vi "Teleop.vi"(10 "Match Info":T2={"Autonomous Elapsed Seconds"=0.0, "TeleOp Elapsed Seconds"=0.0, "Disabled Elapsed Seconds"=0.0, "Visited Autonomous"=FALSE, "Visited TeleOp"=FALSE, "Visited Disabled"=FALSE, "Autonomous Settings"={"Autonomous Style"=enum."Independent", "VI Refnum"=refnum}}, 11 "Call Context":T3) -> ()   [LabVIEW 2020]
doc: "This VI is called for each TeleOp packet received from the DS where the robot is not disabled. It is often used to read from the joysticks and update I/O or to update setpoints for timed control loops. It should complete and return within 20 milliseconds or it may miss DS packets."
uses:
  <vilib>/Rock Robotics/WPI/DriverStation/WPI_DriverStationDerivedRobotMode.ctl
  <vilib>/Rock Robotics/WPI/DriverStation/WPI_DriverStationMatch Info.ctl
  <vilib>/Rock Robotics/WPI/Solenoid/WPI_SolenoidValue.ctl
  <vilib>/Rock Robotics/WPI/ThirdParty/Phoenix-LabVIEW/Motor Controller/Controls/CTRE_Phoenix_MotorControl_ControlMode.ctl
  <vilib>/Rock Robotics/WPI/Utilities/WPI_GetSetVariantRefNum.vi
  <vilib>/Rock Robotics/Network Tables/NT Write Boolean Array.vi
  <vilib>/Rock Robotics/Network Tables/NT Write Numeric Array.vi
  <vilib>/Rock Robotics/Network Tables/NT Read Boolean.vi
  <vilib>/Rock Robotics/Network Tables/NT Read Number.vi
  <vilib>/Rock Robotics/WPI/Solenoid/WPI_SolenoidSetEnum.vi
  Robot Global Data.vi
panel:
  out "start_control_panel":bool
  out "control_panel_arm_output":dbl
  out "encoder_setpoint":dbl=1409.0
  out "intake_motor_output":dbl
  out "control_arm_cylinder":T1
  out "intake_cylinder":T1
  out "climb_cylinder":T1
  out "Sample Slider 0":dbl(slide) scale=0.0..5.0
  out "Sample Boolean 1":bool
  out "Sample Boolean 0":bool
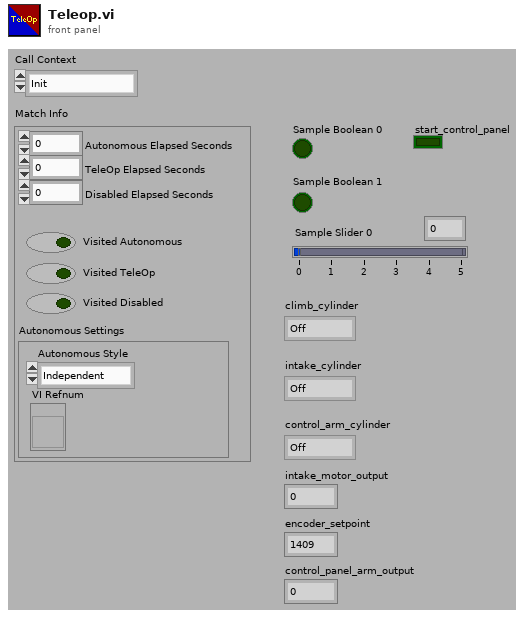
[diagram p1: front panel]
types:
  T1 = typedef "WPI_SolenoidValue.ctl" = enum16{"Off", "On", "Forward", "Reverse"}
  T2 = typedef "WPI_DriverStationMatch Info.ctl" = cluster{"Autonomous Elapsed Seconds":dbl, "TeleOp Elapsed Seconds":dbl, "Disabled Elapsed Seconds":dbl, "Visited Autonomous":bool, "Visited TeleOp":bool, "Visited Disabled":bool, "Autonomous Settings":cluster{"Autonomous Style":enum16{"Iterative", "Independent"}, "VI Refnum":refnum<vi>}}
  T3 = typedef "WPI_DriverStationDerivedRobotMode.ctl" = enum16{"Init", "Execute", "Stop"}
  T4 = typedef "CTRE_Phoenix_MotorControl_ControlMode.ctl" = u16
  T5 = typedef "WPI_JoystickDevRef.ctl" = cluster{"Device":T6}
  T6 = typedef "WPI_JoystickDeviceEnum.ctl" = enum16{"USB 0", "USB 1", "USB 2", "USB 3", "USB 4", "USB 5"}
  T7 = typedef "WPI_RobotDriveDevRef.ctl" = cluster{"DevStatus":errorcluster, "Motors[]":T8[], "Square Inputs":bool, "Max Output":dbl}
  T8 = typedef "WPI_MotorControlDeviceRef.ctl" = cluster{"DeviceStatus":errorcluster, "Type":T9, "PWM":cluster{"PWM Channel":T10, "DeadBand":T11}, "CAN":cluster{"Device Number":u8, "SetOutput VI Ref":variant, "GetOutput VI Ref":variant, "Enable VI Ref":variant, "Disable VI Ref":variant, "Data":variant}, "Invert":bool, "DIO PWM":cluster{"PWM \"Enable\" Channel":T10, "DIOChannel":T12, "PWM Rate":dbl}}
  T9 = typedef "WPI_MotorControlType.ctl" = enum16{"PWM", "CAN", "DIO PWM"}
  T10 = typedef "FPGA_DIOPWMChannel.ctl" = enum8{"PWM 0", "PWM 1", "PWM 2", "PWM 3", "PWM 4", "PWM 5", "PWM 6", "PWM 7", "PWM 8", "PWM 9", "PWM MXP 0", "PWM MXP 1", "PWM MXP 2", "PWM MXP 3", "PWM MXP 4", "PWM MXP 5", "PWM MXP 6", "PWM MXP 7", "PWM MXP 8", "PWM MXP 9", "Invalid"}
  T11 = typedef "WPI_PWMDeadband.ctl" = cluster{"Name":string, "maxPositivePwm":i32, "minPositivePwm":i32, "centerPwm":i32, "maxNegativePwm":i32, "minNegativePwm":i32, "angularRange":u16}
  T12 = typedef "FPGA_DIOChannel.ctl" = enum8{"DIO 0", "DIO 1", "DIO 2", "DIO 3", "DIO 4", "DIO 5", "DIO 6", "DIO 7", "DIO 8", "DIO 9", "DIO MXP 0", "DIO MXP 1", "DIO MXP 2", "DIO MXP 3", "DIO MXP 4", "DIO MXP 5", "DIO MXP 6", "DIO MXP 7", "DIO MXP 8", "DIO MXP 9", "DIO MXP 10", "DIO MXP 11", "DIO MXP 12", "DIO MXP 13", "DIO MXP 14", "DIO MXP 15", "SPI Port CS1", "SPI Port CS2", "SPI Port CS3", "SPI Port MISO", "SPI Port MOSI", "Invalid"}
  T13 = typedef "WPI_SolenoidDevRef.ctl" = cluster{"DevStatus":errorcluster, "Pneumatics Control Module":u8, "Forward Solenoid Channel":T14, "Reverse Solenoid Channel":T14}
  T14 = typedef "WPI_SolenoidChannel.ctl" = enum8{"Solenoid 0", "Solenoid 1", "Solenoid 2", "Solenoid 3", "Solenoid 4", "Solenoid 5", "Solenoid 6", "Solenoid 7", "Solenoid 8", "Solenoid 9", "Solenoid 10", "Solenoid 11", "Solenoid 12", "Solenoid 13", "Solenoid 14", "Solenoid 15", "Invalid"}
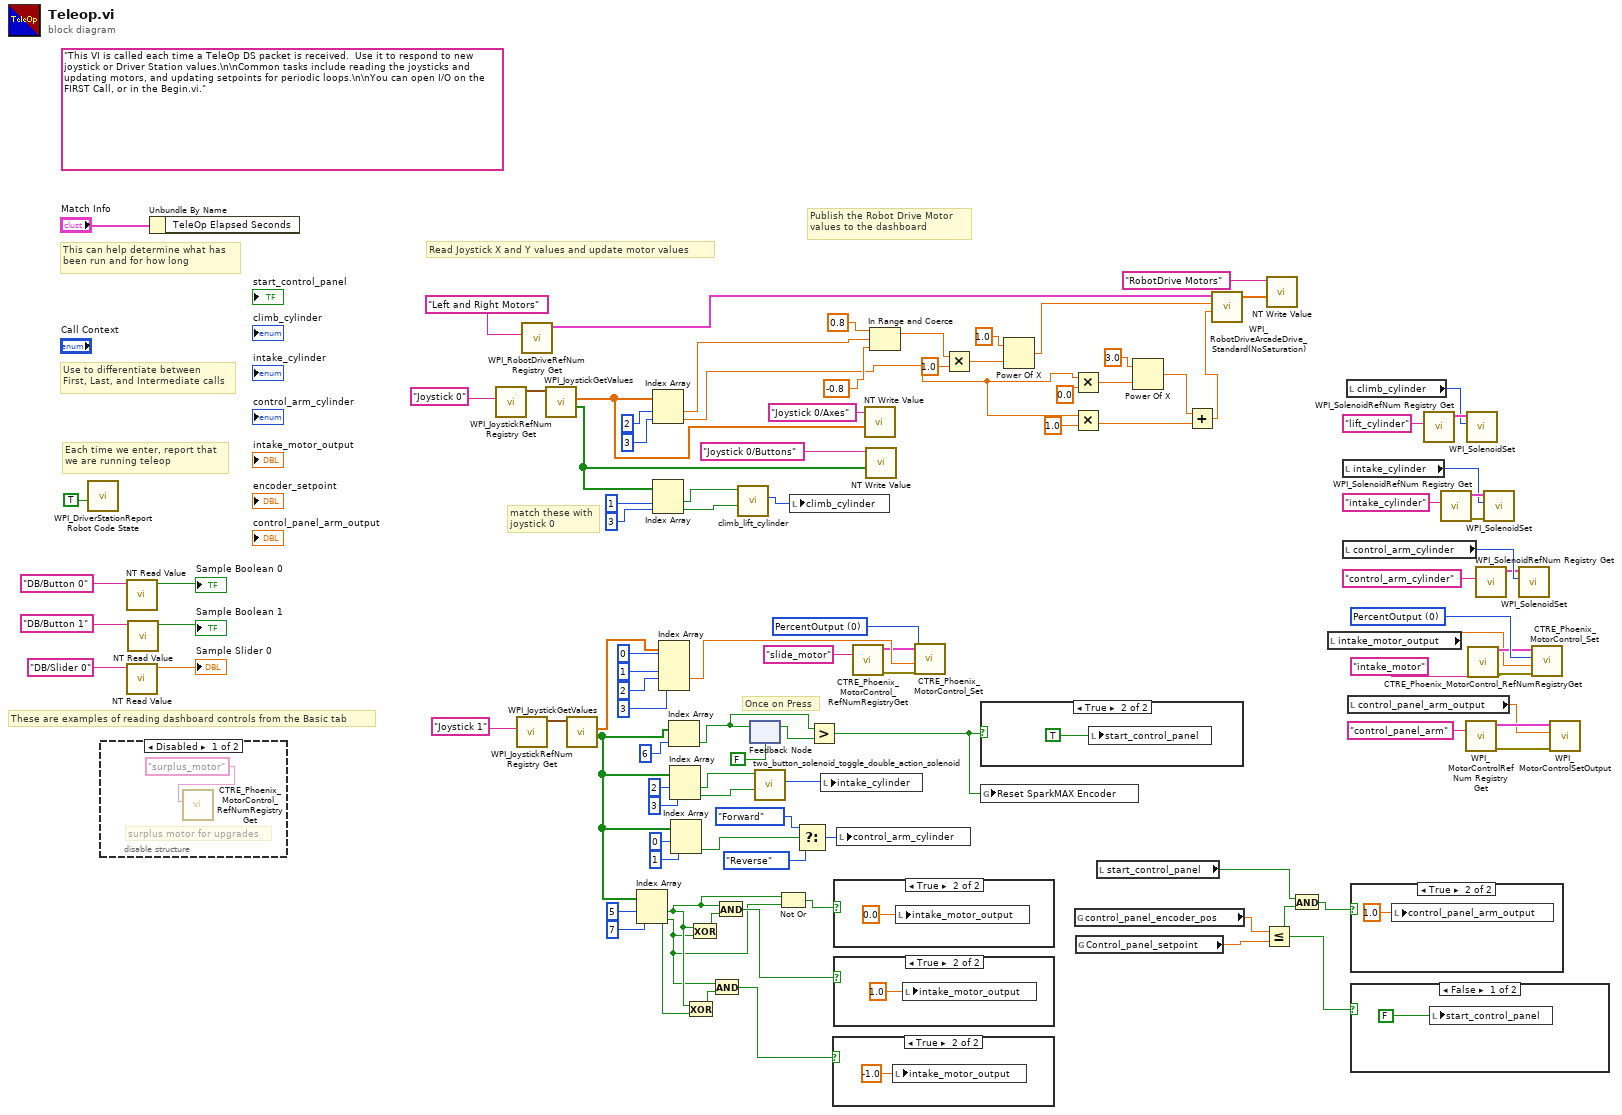
[diagram p0: block diagram]
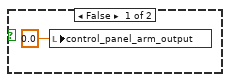
[diagram p4: hidden frame]
diagram:
  w48 = T4 0 items=["PercentOutput"=0, "Position"=1, "Velocity"=2, "Current"=3, "Follower"=5, "MotionProfile"=6, "MotionMagic"=7, "MotionProfileArc"=10, "Disabled"=15] ("Control Mode")
  w49 = T4 0 items=["PercentOutput"=0, "Position"=1, "Velocity"=2, "Current"=3, "Follower"=5, "MotionProfile"=6, "MotionMagic"=7, "MotionProfileArc"=10, "Disabled"=15] ("Control Mode")
  (unwired) "This VI is called each time a TeleOp DS packet is received.  Use it to respond to new joystick or Driver Station values.\n\nCommon tasks include reading the joysticks and updating motors, and updating setpoints for periodic loops.\n\nYou can open I/O on the FIRST Call, or in the Begin.vi."
  # "Once on Press"
  # "match these with\njoystick 0"
  # "These are examples of reading dashboard controls from the Basic tab"
  # "Publish the Robot Drive Motor\nvalues to the dashboard"
  # "Each time we enter, report that\nwe are running teleop"
  # "Use to differentiate between\nFirst, Last, and Intermediate calls"
  # "This can help determine what has\nbeen run and for how long"
  # "Read Joystick X and Y values and update motor values"
  n1 = call <vilib>:"WPI_DriverStationReport Robot Code State.vi"("TeleOp"=TRUE ("Autonomous")) -> ()  [unwired: 10 in, 1 out]
  n2 = disable-structure shown="Disabled" {
    frame Disabled {
      # "surplus motor for upgrades"
      n3 = call <vilib>:"CTRE_Phoenix_MotorControl_RefNumRegistryGet.vi"("refnum name"="surplus_motor") -> ()  [unwired: 9 in, 2 out]
    }
    frame Enabled {
    }
  }
  n4 = call-poly <vilib>:"NT Read Value.vi"("Name"="DB/Button 0" ("refnum name")) -> ("Boolean"=→"Sample Boolean 0":bool)  [unwired: 9 in, 1 out]
  n5 = call-poly <vilib>:"NT Read Value.vi"("Name"="DB/Slider 0" ("refnum name")) -> ("Numeric"=→"Sample Slider 0":dbl)  [unwired: 9 in, 1 out]
  n6 = call-poly <vilib>:"NT Read Value.vi"("Name"="DB/Button 1" ("refnum name")) -> ("Boolean"=→"Sample Boolean 1":bool)  [unwired: 9 in, 1 out]
  n7 = Unbundle By Name("Match Info") -> ()  [unwired: 1 out]
  n8 = call <vilib>:"WPI_JoystickRefNum Registry Get.vi"("refnum name"="Joystick 0") -> ("JoystickDevRef"=w99:T5)  [unwired: 1 in, 9 out]
  n9 = call <vilib>:"WPI_JoystickRefNum Registry Get.vi"("refnum name"="Joystick 1") -> ("JoystickDevRef"=w83:T5)  [unwired: 1 in, 9 out]
  n10 = call <vilib>:"WPI_RobotDriveRefNum Registry Get.vi"("refnum name"="Left and Right Motors") -> ("RobotDriveDevRef"=w101:T7)  [unwired: 1 in, 9 out]
  n11 = call <vilib>:"WPI_JoystickGetValues.vi"("JoystickDevRef"=w99) -> ("Buttons"=w81:bool[], "Axes"=w95:dbl[])  [unwired: 6 in, 3 out]
  n12 = call <vilib>:"WPI_JoystickGetValues.vi"("JoystickDevRef"=w83) -> ("Buttons"=w33:bool[], "Axes"=w84:dbl[])  [unwired: 6 in, 3 out]
  n13 = Index Array(array=w33, index #1=5 ("index"), index #2=7 ("index")) -> (element #1=w40:bool, element #2=w39:bool)
  n14 = Index Array(array=w95, index #1=2 ("index"), index #2=3 ("index")) -> (element #1=w14:dbl, element #2=w2:dbl)
  n15 = Index Array(array=w81, index #1=1 ("index"), index #2=3 ("index")) -> (element #1=w76:bool, element #2=w75:bool)
  n16 = Index Array(array=w84, index #1=0 ("index"), index #2=1 ("index"), index #3=2 ("index"), index #4=3 ("index")) -> (element #3=w56:dbl)  [unwired: 3 out]
  n17 = Index Array(array=w33, index=6) -> (element=w22:bool)
  n18 = Index Array(array=w33, index #1=2 ("index"), index #2=3 ("index")) -> (element #1=w62:bool, element #2=w61:bool)
  n19 = Index Array(array=w33, index #1=0 ("index"), index #2=1 ("index")) -> (element #2=w24:bool)  [unwired: 1 out]
  n20 = Exclusive Or(1:w39, 2:w40) -> (0:w52:bool)
  n21 = Exclusive Or(1:w39, 2:w40) -> (0:w53:bool)
  n22 = And(x=w39, y=w52) -> (x .and. y?=w50:bool)
  n23 = And(x=w40, y=w53) -> (x .and. y?=w51:bool)
  n24 = call "climb_lift_cylinder.vi"("Button A"=w76, "Button B"=w75) -> ("climb_lyft_cylinder"=w29:T1)  [unwired: 8 in]
  n25 = feedback-in #1(w22) -> ()
  n26 = feedback #1(FALSE) -> (w21:bool)
  n27 = call "two_button_solenoid_toggle_double_action_solenoid.vi"("Button A"=w62, "Button B"=w61) -> ("Cylinder_out"=w67:T1)  [unwired: 8 in]
  n28 = Not Or(1:w39, 2:w40) -> (0:w38:bool)
  n29 = local write "climb_cylinder"(w29) -> ()
  n30 = Select(t=WPI_SolenoidValue."Forward" ("Value"), s=w24, f=WPI_SolenoidValue."Reverse" ("Value")) -> (s? t:f=w27:T1)
  n31 = Greater?(x=w22, y=w21) -> (0:w17:bool)
  n32 = local write "intake_cylinder"(w67) -> ()
  n33 = case shown="True" w50 {
    frame False {
    }
    frame True {
      n34 = local write "intake_motor_output"(-1.0) -> ()
    }
  }
  n35 = case shown="True" w38 {
    frame False {
    }
    frame True {
      n36 = local write "intake_motor_output"(0.0) -> ()
    }
  }
  n37 = case shown="True" w51 {
    frame False {
    }
    frame True {
      n38 = local write "intake_motor_output"(1.0) -> ()
    }
  }
  n39 = local write "control_arm_cylinder"(w27) -> ()
  n40 = call <vilib>:"CTRE_Phoenix_MotorControl_RefNumRegistryGet.vi"("refnum name"="slide_motor") -> ("error out"=w45:errorcluster, "PhoenixMotorControlDevRef"=w46:T8)  [unwired: 9 in]
  n41 = call-poly <vilib>:"NT Write Value.vi"("Numeric Array"=w95, "Name"="Joystick 0/Axes") -> ()  [unwired: 9 in, 1 out]
  n42 = call-poly <vilib>:"NT Write Value.vi"("Boolean Array"=w81, "Name"="Joystick 0/Buttons") -> ()  [unwired: 9 in, 1 out]
  n43 = In Range and Coerce(upper limit=0.8, x=w14, lower limit=-0.8) -> (coerced(x)=w11:dbl)  [unwired: 1 out]
  n44 = call <vilib>:"CTRE_Phoenix_MotorControl_Set.vi"("error in (no error)"=w45, "Output"=w56, "Control Mode"=w48, "PhoenixMotorControlDevRef"=w46) -> ()  [unwired: 6 in, 2 out]
  n45 = Multiply(x=w11, y=1.0) -> (x*y=w10:dbl)
  n46 = case shown="True" w17 {
    frame False {
    }
    frame True {
      n47 = local write "start_control_panel"(TRUE) -> ()
    }
  }
  n48 = global write "Robot Global Data.vi" "Reset SparkMAX Encoder"(w17) -> ()
  n49 = Power Of X(1:w10, 2:1.0 ("y")) -> (0:w12:dbl)
  n50 = Multiply(x=w2, y=0.0) -> (x*y=w7:dbl)
  n51 = Multiply(x=w2, y=1.0) -> (x*y=w3:dbl)
  n52 = global read "Robot Global Data.vi" "control_panel_encoder_pos"() -> (w34:dbl)
  n53 = global read "Robot Global Data.vi" "Control_panel_setpoint"() -> (w19:dbl)
  n54 = local read "start_control_panel"() -> (w18:bool)
  n55 = Power Of X(1:w7, 2:3.0 ("y")) -> (0:w4:dbl)
  n56 = Add(x=w4, y=w3) -> (x+y=w5:dbl)
  n57 = call <vilib>:"WPI_RobotDriveArcadeDrive_Standard(NoSaturation).vi"("Y axis value"=w5, "X axis value"=w12, "RobotDriveDevRef"=w101) -> ("Motor Values"=w88:dbl[])  [unwired: 1 in, 7 out]
  n58 = Less Or Equal?(x=w34, y=w19) -> (x <= y?=w20:bool)
  n59 = call-poly <vilib>:"NT Write Value.vi"("Numeric Array"=w88, "Name"="RobotDrive Motors") -> ()  [unwired: 9 in, 1 out]
  n60 = And(x=w18, y=w20) -> (x .and. y?=w30:bool)
  n61 = local read "intake_motor_output"() -> (w41:dbl)
  n62 = local read "intake_cylinder"() -> (w70:T1)
  n63 = local read "control_arm_cylinder"() -> (w69:T1)
  n64 = local read "climb_cylinder"() -> (w28:T1)
  n65 = local read "control_panel_arm_output"() -> (w31:dbl)
  n66 = case shown="True" w30 {
    frame False {
      n67 = local write "control_panel_arm_output"(0.0 ("control_panel_arm_output")) -> ()
    }
    frame True {
      n68 = local write "control_panel_arm_output"(1.0 ("control_panel_arm_output")) -> ()
    }
  }
  n69 = case shown="False" w20 {
    frame False {
      n70 = local write "start_control_panel"(FALSE) -> ()
    }
    frame True {
    }
  }
  n71 = call <vilib>:"WPI_SolenoidRefNum Registry Get.vi"("refnum name"="lift_cylinder") -> ("SolenoidDevRef"=w77:T13)  [unwired: 9 in, 1 out]
  n72 = call <vilib>:"WPI_SolenoidRefNum Registry Get.vi"("refnum name"="intake_cylinder") -> ("error out"=w72:errorcluster, "SolenoidDevRef"=w71:T13)  [unwired: 9 in]
  n73 = call <vilib>:"WPI_MotorControlRefNum Registry Get.vi"("refnum name"="control_panel_arm") -> ("error out"=w36:errorcluster, "MotorControlDevRef"=w37:T8)  [unwired: 9 in]
  n74 = call-poly <vilib>:"WPI_SolenoidSet.vi"("Value"=w28, "SolenoidDevRef"=w77) -> ()  [unwired: 8 in, 2 out]
  n75 = call <vilib>:"CTRE_Phoenix_MotorControl_RefNumRegistryGet.vi"("refnum name"="intake_motor") -> ("error out"=w43:errorcluster, "PhoenixMotorControlDevRef"=w44:T8)  [unwired: 9 in]
  n76 = call <vilib>:"WPI_SolenoidRefNum Registry Get.vi"("refnum name"="control_arm_cylinder") -> ("SolenoidDevRef"=w68:T13)  [unwired: 9 in, 1 out]
  n77 = call-poly <vilib>:"WPI_SolenoidSet.vi"("error in (no error)"=w72, "Value"=w70, "SolenoidDevRef"=w71) -> ()  [unwired: 7 in, 2 out]
  n78 = call-poly <vilib>:"WPI_SolenoidSet.vi"("Value"=w69, "SolenoidDevRef"=w68) -> ()  [unwired: 8 in, 2 out]
  n79 = call <vilib>:"CTRE_Phoenix_MotorControl_Set.vi"("error in (no error)"=w43, "Output"=w41, "Control Mode"=w49, "PhoenixMotorControlDevRef"=w44) -> ()  [unwired: 6 in, 2 out]
  n80 = call <vilib>:"WPI_MotorControlSetOutput.vi"("error in (no error)"=w36, "Output"=w31, "MotorControlDevRef"=w37) -> ()  [unwired: 6 in, 3 out]
